vi "NI6071E.ConfigureDAQ.vi"(0 "i ref in":refnum<vi>, 1 "Use attribute data (f)":bool, 2 "NI6071E Config":T3={"device (1)"=1, "channels (0)"=["0"], "buffer size (1000 scans)"=1000, "[number of buffers] (1)"=1, "measurement mode structure"={"measurement mode"=0, "reserved"=0}, "input limits (no change)"=[], "coupling & input config (no change:0)"=[]} {"measurement mode structure"."measurement mode" items=["no change", "Volts", "Volts RMS", "Ohms", "Diode", "4-wire ohms", "Current", "Current RMS"]; "coupling & input config (no change:0)"."input config (no change:0)" items=["no change", "differential", "ref. single-ended", "non-ref. single-ended", "4-wire"]; "input limits (no change)"."low limit (0.0)" format="%0.2f"; "input limits (no change)"."high limit (0.0)" format="%0.2f"}, 4 "timeout ms (60000)":i32=60000, 5 "error in (no error)":errorcluster) -> (14 "i ref out":refnum<vi>, 19 "error out":errorcluster)   [LabVIEW 2014, in "NI6071E.lvlib"]
uses:
  NI6071E.lvlib
  NI6071EConfig.ctl
  NI6071ECommandCluster.ctl
  NI6071ECommand.ctl
panel:
  in  "NI6071E Command":T1=enum."ConfigureDAQ"
  in  "NI6071E Command Cluster":T2
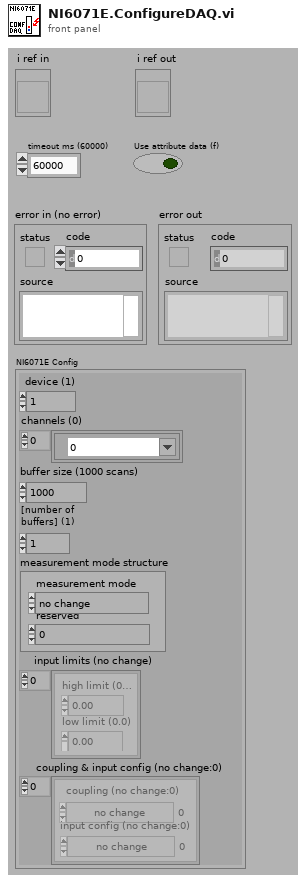
[diagram p1: front panel]
types:
  T1 = typedef "NI6071E.lvlib/NI6071ECommand.ctl" = enum16{"Ping", "Reset", "ConfigureDAQ", "StartDAQ", "StopDAQ", "GetDAQStatus", "ReadData", "SaveData", "CloseConnection"}
  T2 = typedef "NI6071E.lvlib/NI6071ECommandCluster.ctl" = cluster{"Command":string, "Data":string, "error out":errorcluster}
  T3 = typedef "NI6071E.lvlib/NI6071EConfig.ctl" = cluster{"device (1)":i16, "channels (0)":tag[], "buffer size (1000 scans)":i32, "[number of buffers] (1)":i32, "measurement mode structure":cluster{"measurement mode":u16, "reserved":u32}, "input limits (no change)":cluster{"high limit (0.0)":sgl, "low limit (0.0)":sgl}[], "coupling & input config (no change:0)":cluster{"coupling (no change:0)":enum16{"no change", "DC", "AC", "GND", "internal ref."}, "input config (no change:0)":u16}[]}
  T4 = typedef "NI6071E.lvlib/NI6071E.i attribute.ctl" = cluster{"NI6071E Server":string, "Port":u16, "NI6071E Config":T3, "NI6071E Start":T5, "Waveforms":waveform(dbl)[], "RT Error":errorcluster, "NI6071E Read":T6, "connection ID":refnum<k5>, "DAQ Status":string, "device (1)":i16, "DAQ Status Service ID":i32}
  T5 = typedef "NI6071E.lvlib/NI6071EStart.ctl" = cluster{"scan rate (40000 scans/sec)":sgl, "trigger type (analog)":enum16{"no trigger", "analog", "digital A", "digital A & B", "scan clock gate"}, "edge or slope \n(rising)":enum16{"no change", "rising", "falling"}, "number of buffers to acquire (1)":i32, "analog chan (PFI0) & level (2.00)":cluster{"trigger channel (empty)":string, "level (0.0)":sgl}, "[additional trig params]":cluster{"hysteresis (0.0)":sgl, "coupling (no change:0)":enum16{"no change", "DC", "AC"}, "delay (0 sec)":sgl, "skip count (0)":i32, "time limit (0 sec)":sgl}}
  T6 = typedef "NI6071E.lvlib/NI6071ERead.ctl" = cluster{"time limit in sec (-1:auto calculate)":sgl, "number of scans to read (-1:all)":i32}
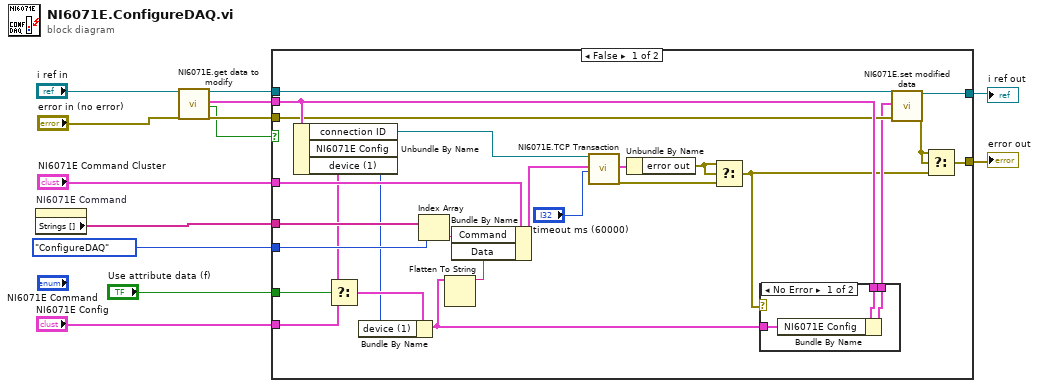
[diagram p0: block diagram]
diagram:
  n1 = property on="NI6071E Command" class="Enum (strict)"() -> ("Strings []"=w5:string[])  [unwired: 2 in, 2 out]
  n2 = call "NI6071E.get data to modify.vi"("i ref in"="i ref in", "error in (no error)"="error in (no error)") -> ("i ref out"=w9:refnum<vi>, "i attribute"=w11:T4, "timed out"=w1:bool, "error out"=w10:errorcluster)  [unwired: 14 in]
  n3 = case shown="False" w1 {
    tunnel: w11 -> [w38 _]
    tunnel: w10 -> [w37 w43]
    tunnel: w9 -> [w36 w44]
    tunnel: [w35 w44] -> w8
    tunnel: [w33 w43] -> w7
    tunnel: "NI6071E Command Cluster" -> [w30 _]
    tunnel: w5 -> [w28 _]
    tunnel: NI6071ECommand."ConfigureDAQ" ("PPMA Command") -> [w27 _]
    tunnel: "NI6071E Config" -> [w18 _]
    tunnel: "Use attribute data (f)" -> [w17 _]
    frame False {
      n4 = Unbundle By Name(w38) -> ("connection ID"=w31:refnum<k5>, "NI6071E Config"=w19:T3, "device (1)"=w14:i16)
      n5 = Select(t=w19, s=w17, f=w18) -> (s? t:f=w16:T3)
      n6 = Bundle By Name(cluster=w16, "device (1)"=w14) -> (w15:T3)
      n7 = Index Array(array=w28, index=w27) -> (element=w26:string)
      n8 = Flatten To String(anything=w15) -> (data string=w25:string)  [unwired: 3 in, 2 out]
      n9 = Bundle By Name(cluster=w30, "Command"=w26, "Data"=w25) -> (w29:T2)
      n10 = call "NI6071E.TCP Transaction.vi"("connection ID in"=w31, "NI6071E Command Cluster"=w29, "timeout ms (25000)"="timeout ms (60000)") -> ("NI6071E Response"=w23:T2, "error out"=w21:errorcluster)  [unwired: 14 in, 1 out]
      n11 = Unbundle By Name(w23) -> ("error out"=w22:errorcluster)
      n12 = Select(t=w22, s=w22, f=w21) -> (s? t:f=w20:errorcluster)
      n13 = case shown="No Error" w20 {
        tunnel: w38 -> [w41 w42]
        tunnel: [w40 w42] -> w32
        tunnel: w15 -> [w39 _]
        frame No Error {
          n14 = Bundle By Name(cluster=w41, "NI6071E Config"=w39) -> (w40:T4)
        }
        frame Error {
        }
      }
      n15 = call "NI6071E.set modified data.vi"("i ref in"=w36, "i attribute"=w32, "error in (no error)"=w37) -> ("i ref out"=w35:refnum<vi>, "error out"=w34:errorcluster)  [unwired: 15 in]
      n16 = Select(t=w34, s=w34, f=w20) -> (s? t:f=w33:errorcluster)
    }
    frame True {
    }
  }
  "i ref out" <- w8
  "error out" <- w7
